vi "niFpgaBacklashTemplate.vi"(0 "deadband":fxp<+,15,15>, 1 "reset":bool, 2 "input":fxp<+/-,16,16>, 3 "initial output":fxp<+/-,16,16>) -> (7 "output":fxp<+/-,16,16>)   [LabVIEW 2017]
doc: "Implements a backlash or deadband function. <B>output</B> does not change until <B>input</B> differs from the previous <B>output</B> by at least half of <B>deadband</B>. The data type you wire to <B>input</B> determines the <B>output</B> data type."
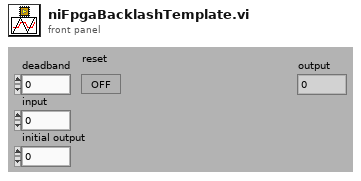
[diagram p1: front panel]
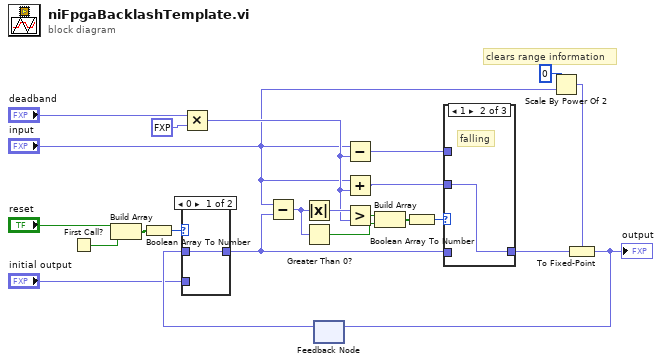
[diagram p0: block diagram]
diagram:
  # "clears range information"
  n1 = First Call?() -> (First Call?: T/F=w21:bool)
  n2 = Build Array("reset", w21) -> (w18:bool[])
  n3 = Boolean Array To Number(Boolean array=w18) -> (number=w19:u8)
  n4 = Multiply(x="deadband", y=fxp<+,1,0> 0.5) -> (x*y=w5:fxp<+,15,14>)
  n5 = feedback #1() -> (w20:fxp<+/-,16,16>)  [unwired: 1 in]
  n6 = case shown="0" w19 {
    tunnel: w20 -> [w24 _]
    tunnel: [w24 w25] -> w11
    tunnel: "initial output" -> [_ w25]
    frame 0 {
    }
    frame Default {
    }
  }
  n7 = Subtract(x="input", y=w11) -> (x-y=w22:fxp<+/-,17,17>)
  n8 = Absolute Value(x=w22) -> (abs(x)=w23:fxp<+,16,16>)
  n9 = Greater Than 0?(x=w22) -> (x > 0?=w14:bool)
  n10 = Subtract(x="input", y=w5) -> (x-y=w17:fxp<+/-,18,17>)
  n11 = Add(x="input", y=w5) -> (x+y=w16:fxp<+/-,18,17>)
  n12 = Greater?(x=w23, y=w5) -> (0:w15:bool)
  n13 = Build Array(w15, w14) -> (w12:bool[])
  n14 = Boolean Array To Number(Boolean array=w12) -> (number=w13:u8)
  n15 = case shown="1" w13 {
    tunnel: w17 -> [_ _ w28]
    tunnel: w16 -> [_ w27 _]
    tunnel: w11 -> [w26 _ _]
    tunnel: [w26 w27 w28] -> w10
    frame Default {
      # "in \ndeadband"
    }
    frame 1 {
      # "falling"
    }
    frame 3 {
      # "rising"
    }
  }
  n16 = Scale By Power Of 2(n=0, x="input") -> (x*2^n=w1:fxp<+/-,16,16>)
  n17 = To Fixed-Point(fixed-point type=w1, number=w10) -> (fixed-point=w7:fxp<+/-,16,16>)
  "output" <- w7
  n18 = feedback-in #1(w7) -> ()
